vi "DAQ_Accel_Excitation.ch.vi"(10 "channel":T1) -> ()   [LabVIEW 2020]
uses:
  <extravilib>/ChannelInstances/Tag-bool/))Channel.ctl
  <vilib>/Utility/error.llb/DialogType.ctl
  <vilib>/DAQmx/read.llb/DAQmx Read (Analog 1D Wfm NChan NSamp).vi
  <extravilib>/ChannelInstances/Tag-bool/Read With Abort.vi
  <vilib>/DAQmx/create/channels.llb/DAQmx Create Channel (AI-Acceleration-Accelerometer).vi
  <vilib>/DAQmx/configure/timing.llb/DAQmx Timing (Sample Clock).vi
  <vilib>/DAQmx/configure/trigger.llb/DAQmx Start Trigger (Digital Edge).vi
  <vilib>/DAQmx/configure/trigger.llb/DAQmx Start Trigger (Time).vi
  <vilib>/DAQmx/configure/trigger.llb/DAQmx Start Trigger (Analog Edge).vi
  <extravilib>/ChannelInstances/Tag-bool/EndpointRead.vi
  <vilib>/DAQmx/miscellaneous.llb/DAQmx Fill In Error Info.vi
  <resource>/objmgr/daqmx.rc
  <extravilib>/ChannelInstances/Tag-bool.lvlib
panel:
  in  "Trigger Type":T2(tab)
  in  "Digital Start Trigger Edge":i32(ring)=10280 caption="Edge" items=["Rising"=10280, "Falling"=10171]
  in  "Digital Start Trigger Source":tag="/Dev1/PFI0" caption="Source"
  in  "Digital Pause Trigger Pause When":i32(ring)=10192 caption="Pause When" items=["High"=10192, "Low"=10214]
  in  "Digital Pause Trigger Source":tag="/Dev1/PFI0" caption="Source"
  in  "Analog Start Trigger Level":dbl caption="Level" format="%0.2f"
  in  "Analog Start Trigger Hysteresis":dbl caption="Hysteresis" format="%.2f"
  in  "Analog Start Trigger Slope":i32(ring)=10280 caption="Slope" items=["Rising"=10280, "Falling"=10171]
  in  "Analog Start Trigger Source":string="APFI0" caption="Source"
  in  "Analog Pause Trigger Source":string="APFI0" caption="Source"
  in  "Analog Pause Trigger Pause When":i32(ring)=10093 caption="Pause When" items=["Above Level"=10093, "Below Level"=10107]
  in  "Analog Pause Trigger Level":dbl caption="Level" format="%.2f"
  in  "When":timestamp
  in  "Select Time\nManually":bool
  out "Waveform Graph":waveform(dbl)[](graph)
  out "Actual Sample Rate":dbl=1000.0 format="%0.2f"
  # "To enable triggers, select a tab above, and configure the settings.\n\nNot all hardware supports all trigger types. Refer to your device documentation for more information."
  # "This trigger type is not supported in continuous sample timing. \n\nRefer to your device documentation for more information on which triggers are supported."
  # "This trigger type is not supported in continuous sample timing. \n\nRefer to your device documentation for more information on which triggers are supported."
  # "If time is not manually set, task will begin after 10 seconds"
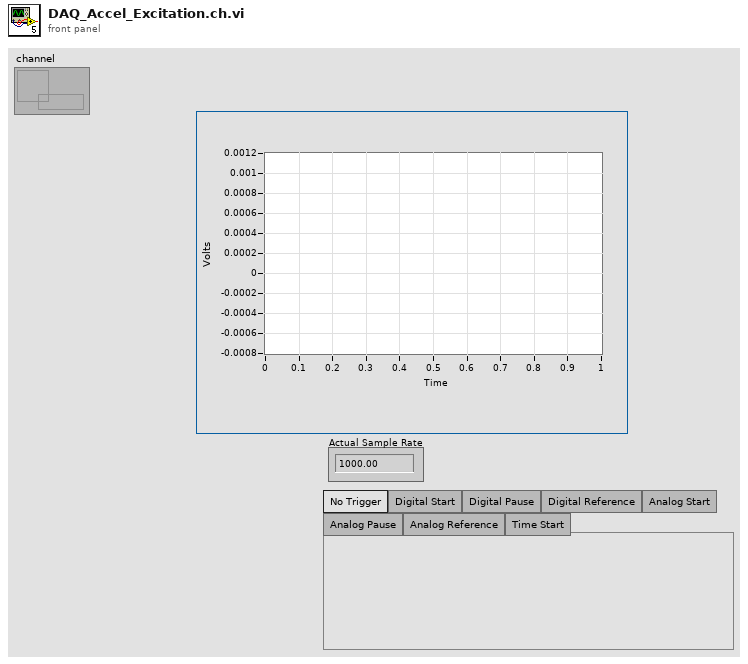
[diagram p1: front panel]
types:
  T1 = typedef "Tag-bool.lvlib/))Channel.ctl" = refnum<queue>
  T2 = enum32{"No Trigger", "Digital Start", "Digital Pause", "Digital Reference", "Analog Start", "Analog Pause", "Analog Reference", "Time Start"}
  T3 = typedef "DialogType.ctl" = u16
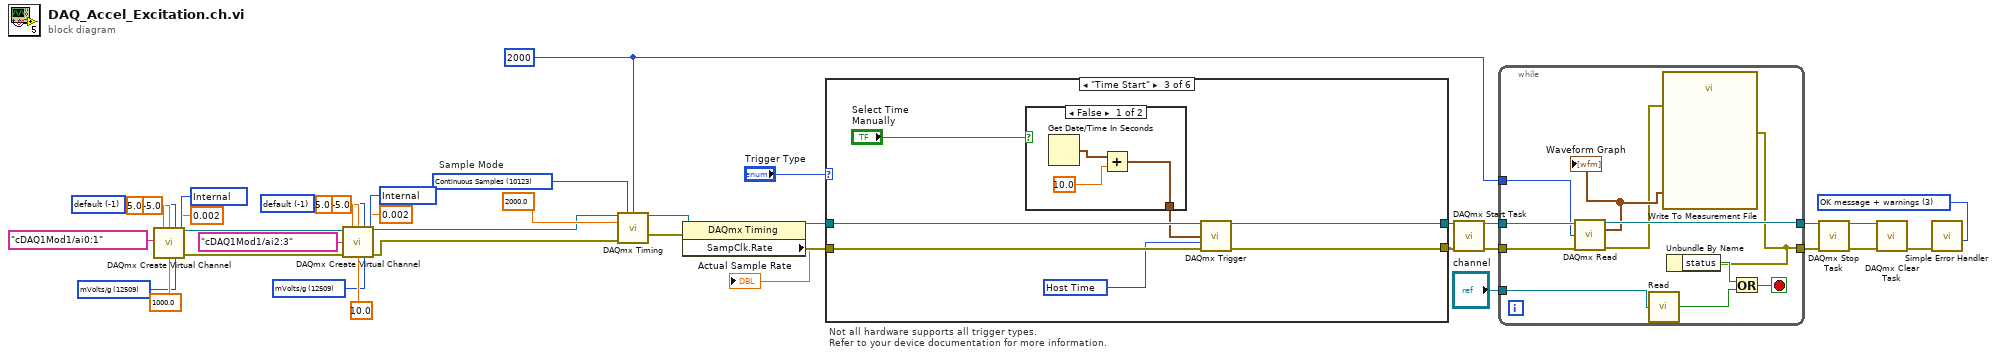
[diagram p0: block diagram]
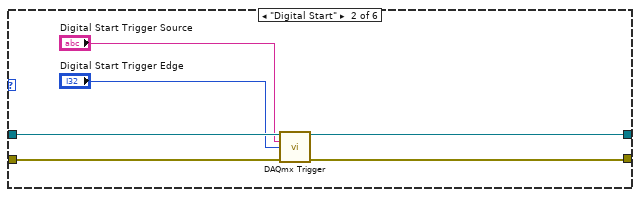
[diagram p3: hidden frame]
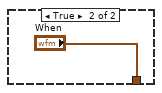
[diagram p4: hidden frame]
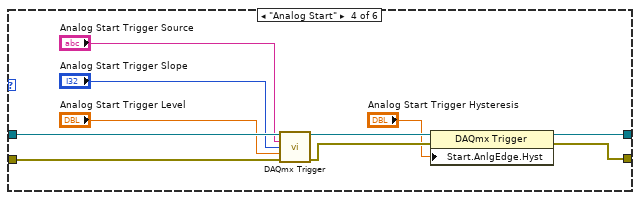
[diagram p5: hidden frame]
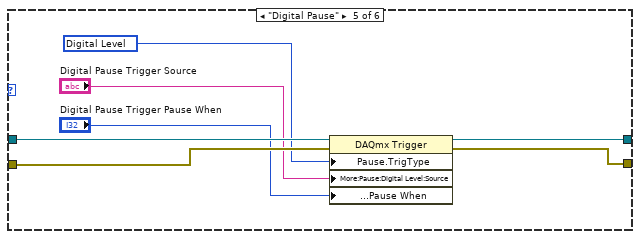
[diagram p6: hidden frame]
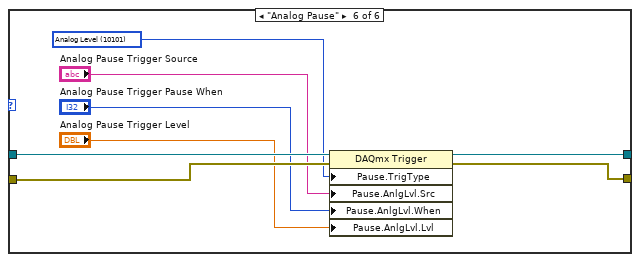
[diagram p7: hidden frame]
diagram:
  w6 = 12509 items=["mVolts/g"=12509, "Volts/g"=12510] ("sensitivity units")
  w7 = 12509 items=["mVolts/g"=12509, "Volts/g"=12510] ("sensitivity units")
  w11 = 10200 items=["Internal"=10200, "External"=10167, "None"=10230] ("current excitation source")
  w12 = -1 items=["default"=-1, "RSE"=10083, "NRSE"=10078, "Differential"=10106, "Pseudodifferential"=12529] ("input terminal configuration")
  w16 = 2000 ("samples per channel")
  w21 = T3 3 items=["no dialog", "OK message", "continue or stop message", "OK message + warnings", "continue/stop + warnings"] ("type of dialog (OK msg:1)")
  w32 = 10123 items=["Finite Samples"=10178, "Continuous Samples"=10123, "Hardware Timed Single Point"=12522]  # Sample Mode
  w36 = 10200 items=["Internal"=10200, "External"=10167, "None"=10230] ("current excitation source")
  w37 = -1 items=["default"=-1, "RSE"=10083, "NRSE"=10078, "Differential"=10106, "Pseudodifferential"=12529] ("input terminal configuration")
  # "Not all hardware supports all trigger types.\nRefer to your device documentation for more information."
  n1 = call-poly <vilib>:"DAQmx Create Virtual Channel.vi"("maximum value"=5.0, "minimum value"=-5.0, "input terminal configuration"=w37, "physical channels"=tag "cDAQ1Mod1/ai0:1", "current excitation source"=w36, "current excitation value"=0.002, "sensitivity"=1000.0, "sensitivity units"=w6) -> ("task out"=w3:refnum<k21>, "error out"=w4:errorcluster)  [unwired: 6 in]
  n2 = call-poly <vilib>:"DAQmx Create Virtual Channel.vi"("task in"=w3, "maximum value"=5.0, "minimum value"=-5.0, "input terminal configuration"=w12, "physical channels"=tag "cDAQ1Mod1/ai2:3", "current excitation source"=w11, "current excitation value"=0.002, "error in"=w4, "sensitivity"=10.0, "sensitivity units"=w7) -> ("task out"=w2:refnum<k21>, "error out"=w5:errorcluster)  [unwired: 4 in]
  n3 = call-poly <vilib>:"DAQmx Timing.vi"("task/channels in"=w2, "sample mode"=w32, "samples per channel"=w16, "rate"=2000.0, "error in"=w5) -> ("task out"=w34:refnum<k21>, "error out"=w33:errorcluster)  [unwired: 9 in]
  n4 = property class="DAQmx Timing"(reference=w34, error in=w33) -> (reference out=w31:refnum<k21>, error out=w30:errorcluster, "SampClk.Rate"=→"Actual Sample Rate":dbl)
  n5 = case shown="\"Time Start\"" "Trigger Type" {
    tunnel: w31 -> [w42 w48 w55 w69 w76 w84]
    tunnel: w30 -> [w41 w47 w54 w68 w73 w81]
    tunnel: [w42 w46 w53 w66 w75 w83] -> w18
    tunnel: [w41 w45 w52 w65 w74 w82] -> w19
    frame "No Trigger", Default {
    }
    frame "Digital Start" {
      n6 = call-poly <vilib>:"DAQmx Trigger.vi"("task/channels in"=w48, "source"="Digital Start Trigger Source", "edge"="Digital Start Trigger Edge", "error in"=w47) -> ("task out"=w46:refnum<k21>, "error out"=w45:errorcluster)  [unwired: 10 in]
    }
    frame "Time Start" {
      w51 = 16126 items=["Host Time"=16126, "I/O Device Time"=16127] ("timescale")
      n7 = case shown="False" "Select Time\nManually" {
        tunnel: [w56 "When"] -> w49
        frame False {
          n8 = Get Date/Time In Seconds() -> (seconds since 1Jan1904=w58:timestamp)
          n9 = Add(x=w58, y=10.0) -> (x+y=w56:timestamp)
        }
        frame True {
        }
      }
      n10 = call-poly <vilib>:"DAQmx Trigger.vi"("task/channels in"=w55, "when"=w49, "timescale"=w51, "error in"=w54) -> ("task out"=w53:refnum<k21>, "error out"=w52:errorcluster)  [unwired: 10 in]
    }
    frame "Analog Start" {
      n11 = call-poly <vilib>:"DAQmx Trigger.vi"("task/channels in"=w69, "source"="Analog Start Trigger Source", "slope"="Analog Start Trigger Slope", "level"="Analog Start Trigger Level", "error in"=w68) -> ("task out"=w64:refnum<k21>, "error out"=w63:errorcluster)  [unwired: 9 in]
      n12 = property class="DAQmx Trigger"(reference=w64, error in=w63, "Start.AnlgEdge.Hyst"="Analog Start Trigger Hysteresis") -> (reference out=w66:refnum<k21>, error out=w65:errorcluster)
    }
    frame "Digital Pause" {
      w72 = 10152 items=["Analog Level"=10101, "Analog Window"=10103, "Digital Level"=10152, "Digital Pattern"=10398, "None"=10230] ("Pause.TrigType")
      n13 = property class="DAQmx Trigger"(reference=w76, error in=w73, "Pause.TrigType"=w72, "More:Pause:Digital Level:Source"="Digital Pause Trigger Source", "More:Pause:Digital Level:Pause When"="Digital Pause Trigger Pause When") -> (reference out=w75:refnum<k21>, error out=w74:errorcluster)
    }
    frame "Analog Pause" {
      w80 = 10101 items=["Analog Level"=10101, "Analog Window"=10103, "Digital Level"=10152, "Digital Pattern"=10398, "None"=10230] ("Pause.TrigType")
      n14 = property class="DAQmx Trigger"(reference=w84, error in=w81, "Pause.TrigType"=w80, "Pause.AnlgLvl.Src"="Analog Pause Trigger Source", "Pause.AnlgLvl.When"="Analog Pause Trigger Pause When", "Pause.AnlgLvl.Lvl"="Analog Pause Trigger Level") -> (reference out=w83:refnum<k21>, error out=w82:errorcluster)
    }
  }
  n15 = call <vilib>:"DAQmx Start Task.vi"("task/channels in"=w18, "error in"=w19) -> ("task out"=w29:refnum<k21>, "error out"=w28:errorcluster)  [unwired: 12 in]
  n16 = while {
    tunnel: w29 -> [w95]
    tunnel: w28 -> [w94]
    tunnel: [w93] -> w25
    tunnel: [w85] -> w24
    tunnel: w16 -> [w90]
    tunnel: "channel" -> [w88]
    stop <- w91 stop-if-true
    n17 = call-poly <vilib>:"DAQmx Read.vi"("task/channels in"=w95, "number of samples per channel"=w90, "error in"=w94) -> ("task out"=w93:refnum<k21>, "data"=w87:waveform(dbl)[], "error out"=w86:errorcluster)  [unwired: 10 in]
    "Waveform Graph" <- w87
    n18 = call <extravilib>:"Read.vi"("channel"=w88) -> ("element"=w89:bool)  [unwired: 1 in, 1 out]
    n19 = call "Write To Measurement File"("Signals"=w87, "error in (no error)"=w86) -> ("error out"=w85:errorcluster)  [unwired: 15 in, 2 out]
    n20 = Unbundle By Name(w85) -> ("status"=w92:bool)
    n21 = Or(x=w92, y=w89) -> (x .or. y?=w91:bool)
  }
  n22 = call <vilib>:"DAQmx Stop Task.vi"("task/channels in"=w25, "error in"=w24) -> ("task out"=w22:refnum<k21>, "error out"=w23:errorcluster)  [unwired: 12 in]
  n23 = call <vilib>:"DAQmx Clear Task.vi"("task in"=w22, "error in"=w23) -> ("error out"=w27:errorcluster)  [unwired: 13 in]
  n24 = call <vilib>:"Simple Error Handler.vi"("type of dialog (OK msg:1)"=w21, "error in (no error)"=w27) -> ()  [unwired: 3 in, 5 out]
